vi "nanocal -- nuclear schottky fit V5.vi"() -> ()   [LabVIEW 2020] (continued)
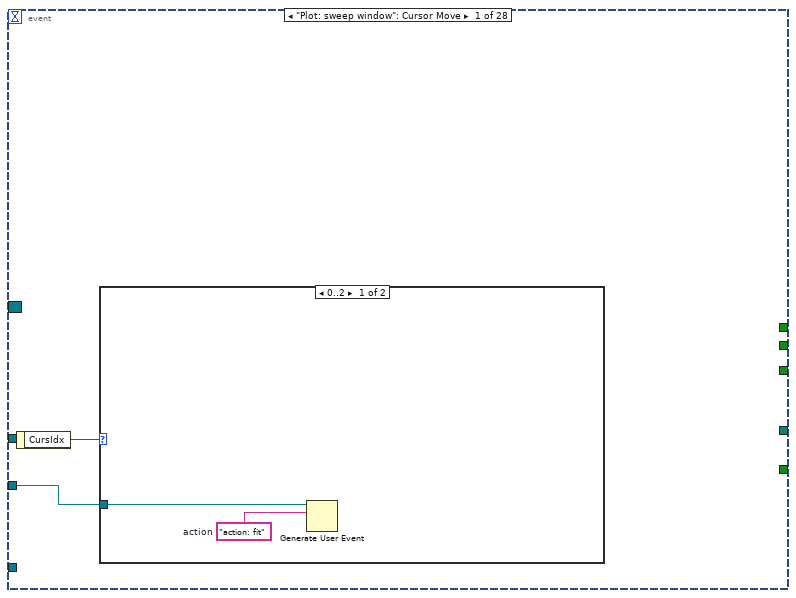
[diagram p2: hidden frame]
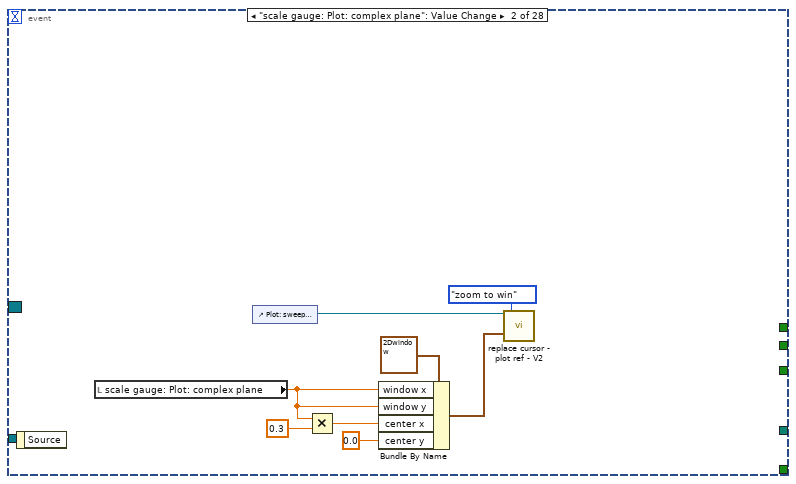
[diagram p4: hidden frame]
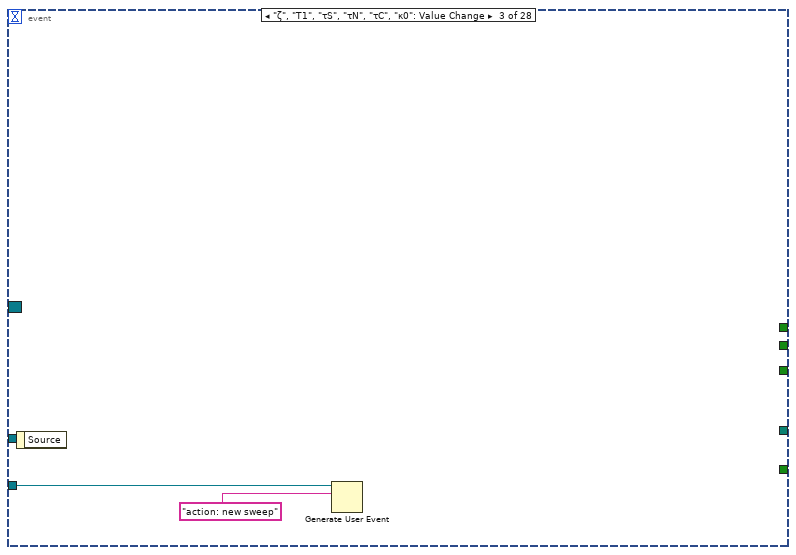
[diagram p5: hidden frame]
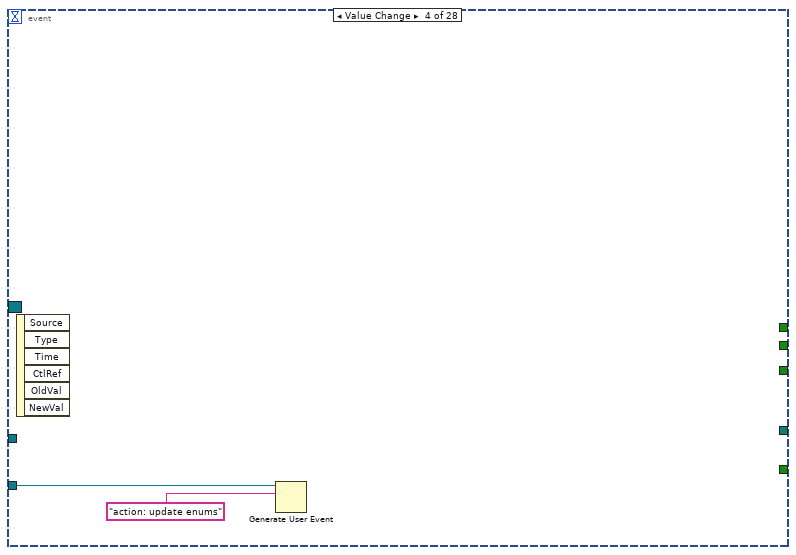
[diagram p6: hidden frame]
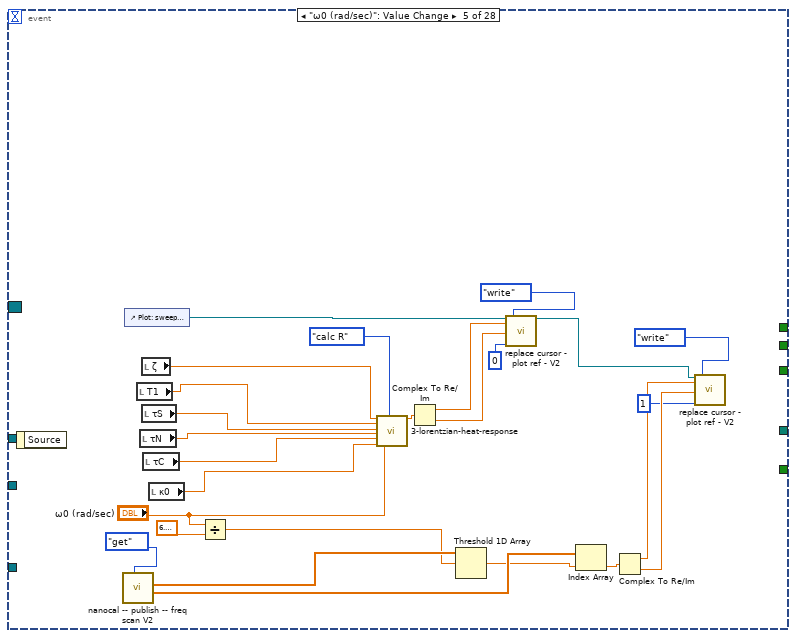
[diagram p7: hidden frame]
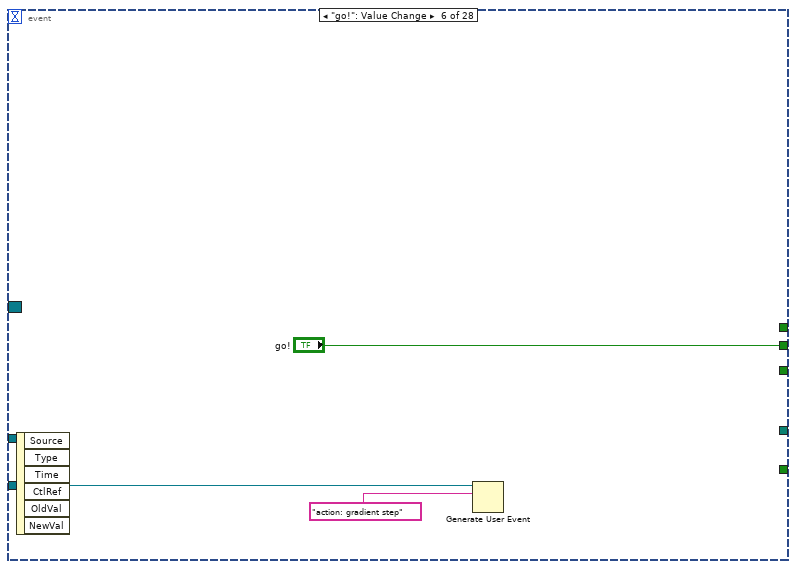
[diagram p8: hidden frame]
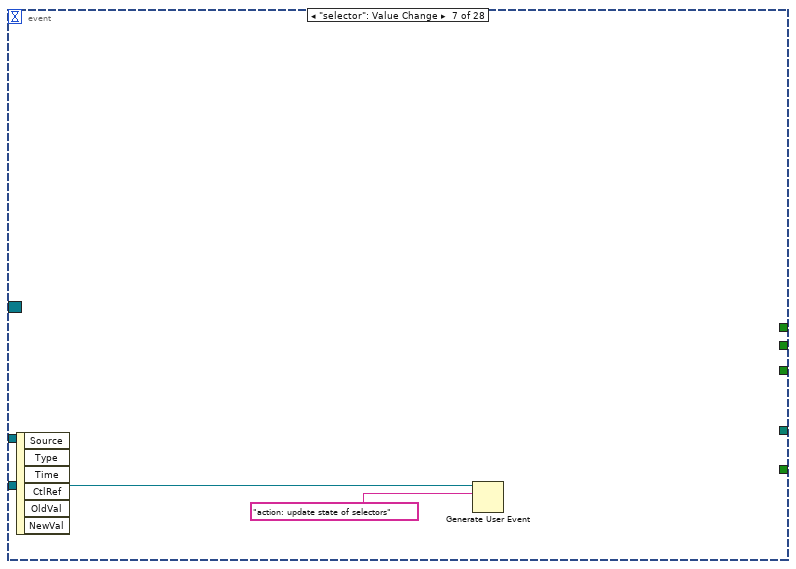
[diagram p9: hidden frame]
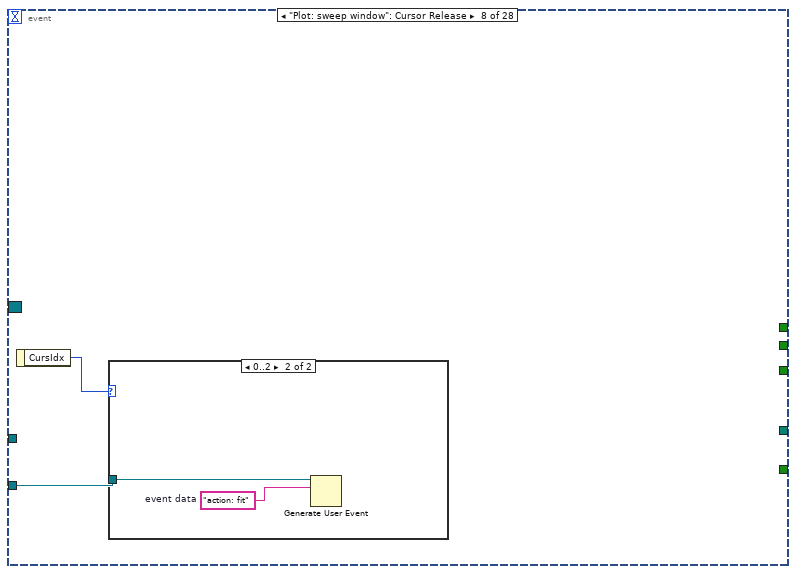
[diagram p10: hidden frame]
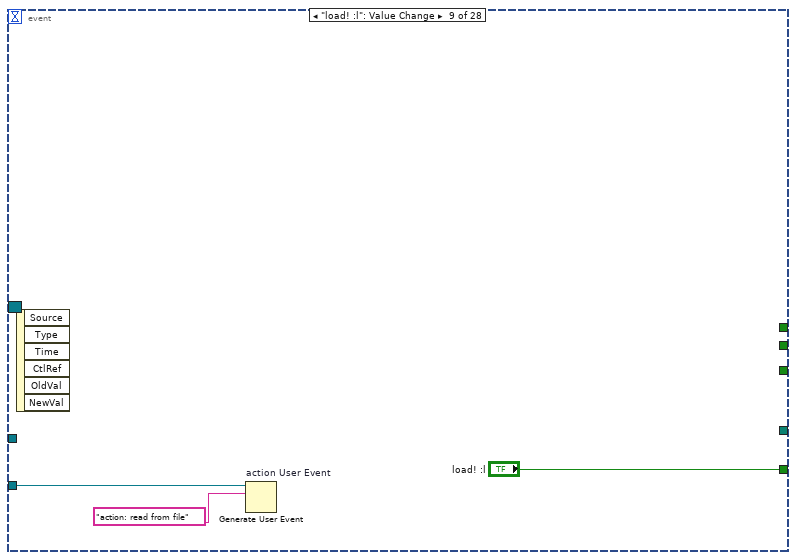
[diagram p12: hidden frame]
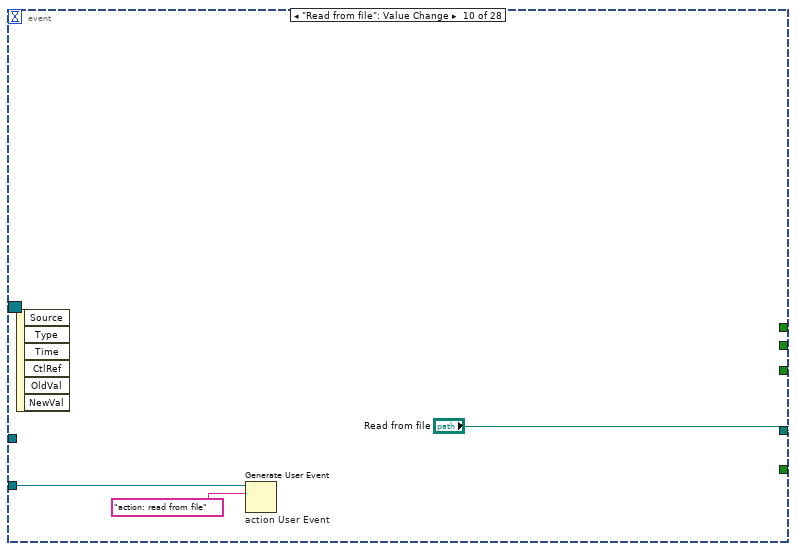
[diagram p13: hidden frame]
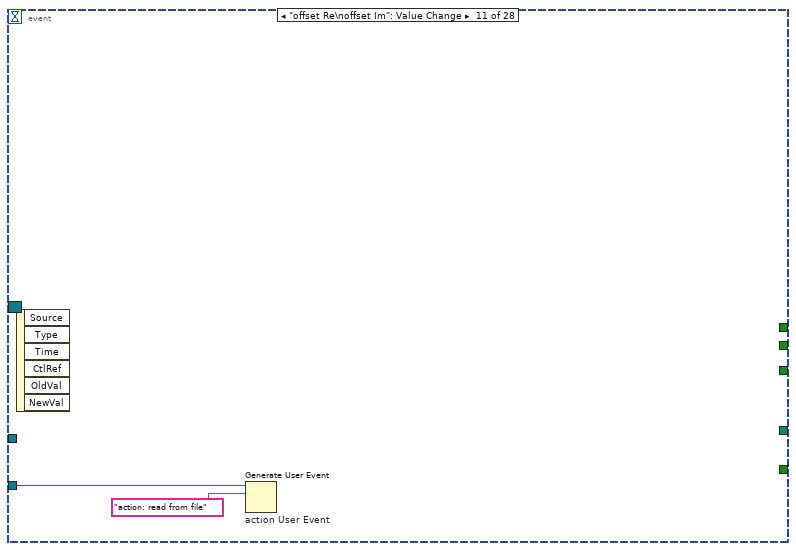
[diagram p14: hidden frame]
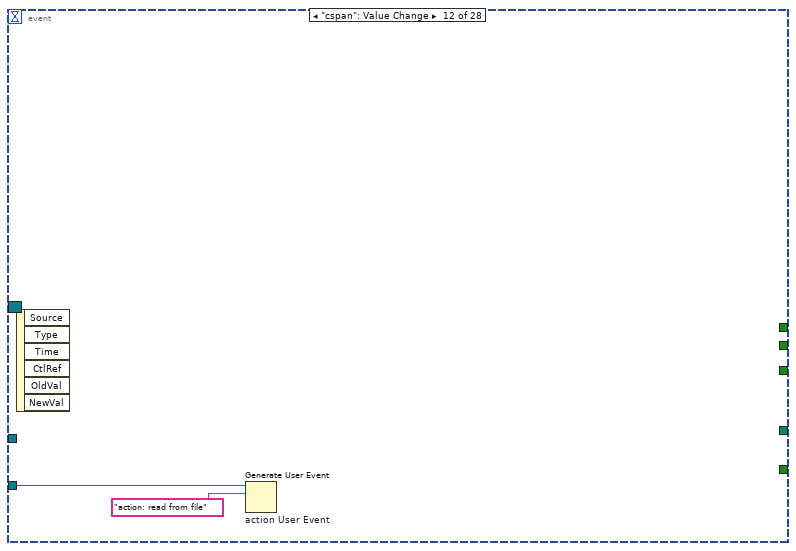
[diagram p15: hidden frame]
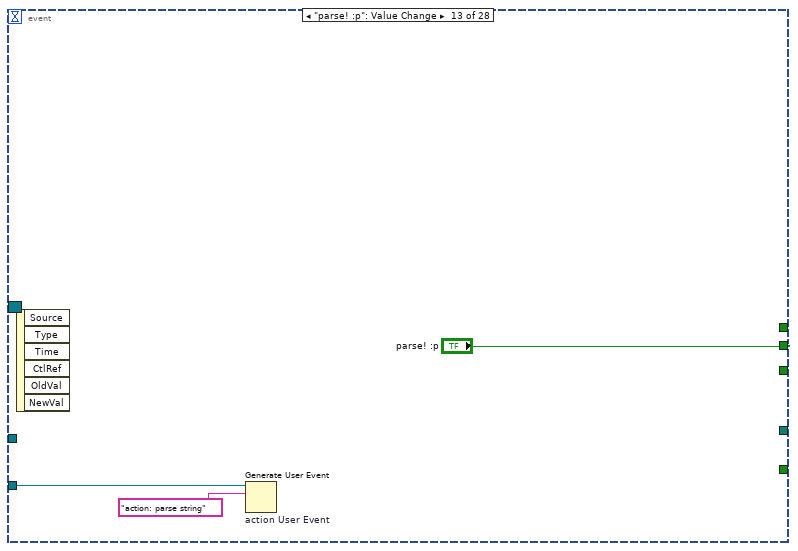
[diagram p16: hidden frame]
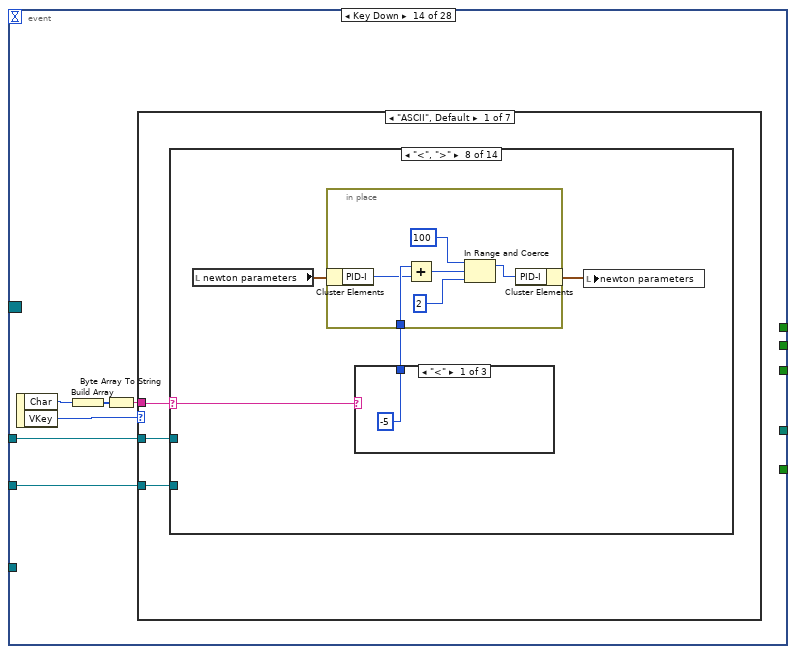
[diagram p17: hidden frame]
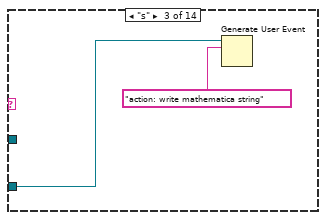
[diagram p20: hidden frame]
              frame "Up", Default {
              }
              frame "Down" {
              }
              frame "Left" {
              }
              frame "Right" {
              }
            }
            n720 = call "replace cursor - plot ref - V2.vi"("Plot ref in"=w1412, "cursor action"=w1414) -> ()  [unwired: 14 in, 4 out]
          }
        }
      }
      event "Plot:  colors": Cursor Move {
        n721 = event-data() -> ("CursIdx"=w1422:i32)  [unwired: 1 in]
        n722 = local read "τS"() -> (w1439:dbl)
        n723 = local read "τN"() -> (w1440:dbl)
        n724 = local read "τC"() -> (w1441:dbl)
        n725 = local read "T1"() -> (w1438:dbl)
        n726 = local read "κ0"() -> (w1442:dbl)
        n727 = local read "ζ"() -> (w1437:dbl)
        n728 = call "replace cursor - plot ref - V2.vi"("Plot ref in"=w1443, "cursor index"=w1422, "cursor action"=cursor_action."read") -> ("read Y"=w1421:dbl)  [unwired: 13 in, 3 out]
        n729 = Build Array(w1437, w1438, w1439, w1440, w1441, w1442) -> (w1424:dbl[])
        n730 = Replace Array Subset(array=w1424, new element=w1421, index=w1422) -> (w1423:dbl[])
        n731 = Index Array(array=w1423, index #1=0 ("index"), index #2=1 ("index"), index #3=2 ("index"), index #4=3 ("index"), index #5=4 ("index"), index #6=5 ("index")) -> (element #1=w1430:dbl, element #2=w1429:dbl, element #3=w1428:dbl, element #4=w1427:dbl, element #5=w1426:dbl, element #6=w1425:dbl)
        n732 = Generate User Event(user event=w1420, event data cluster="action: replot circles" ("event data")) -> ()  [unwired: 2 in, 2 out]
        n733 = local write "τN"(w1427) -> ()
        n734 = local write "τC"(w1426) -> ()
        n735 = local write "τS"(w1428) -> ()
        n736 = local write "κ0"(w1425) -> ()
        n737 = local write "T1"(w1429) -> ()
        n738 = local write "ζ"(w1430) -> ()
      }
      event "pause!": Value Change {
        n739 = event-data() -> ()  [unwired: 1 in, 6 out]
        n740 = local write "newton pause"(TRUE ("newton pause")) -> ()
      }
      event "uco! :u": Value Change {
        n741 = event-data() -> ()  [unwired: 1 in, 1 out]
        n742 = Generate User Event(user event=w1448, event data cluster="ignoreaction: uco" ("event data")) -> ()  [unwired: 2 in, 2 out]
      }
      event "Math→τ! :q": Value Change {
        n743 = event-data() -> ()  [unwired: 1 in, 1 out]
        n744 = Generate User Event(user event=w1451, event data cluster="action: copy from math" ("event data")) -> ()  [unwired: 2 in, 2 out]
      }
      event "load default values": Value Change {
        n745 = event-data() -> ()  [unwired: 1 in, 1 out]
        n746 = Generate User Event(user event=w1453, event data cluster="action: update default values" ("event data")) -> ()  [unwired: 2 in, 2 out]
      }
      event "τ→Math! :p": Value Change {
        n747 = event-data() -> ()  [unwired: 1 in, 1 out]
        n748 = Generate User Event(user event=w1457, event data cluster="action: copy to math" ("event data")) -> ()  [unwired: 2 in, 2 out]
      }
      event "Math→ string OUT! :s": Value Change {
        n749 = event-data() -> ()  [unwired: 1 in, 1 out]
        n750 = Generate User Event(user event=w1460, event data cluster="action: write mathematica string" ("event data")) -> ()  [unwired: 2 in, 2 out]
      }
      event "generate empty string from filelist !": Value Change {
        n751 = event-data() -> ()  [unwired: 1 in, 1 out]
        n752 = Generate User Event(user event=w1463, event data cluster="action: empty string from filelist" ("event data")) -> ()  [unwired: 2 in, 2 out]
      }
      event "string IN → Math!": Value Change {
        n753 = event-data() -> ()  [unwired: 1 in, 1 out]
        n754 = Generate User Event(user event=w1466, event data cluster="action: read mathematica string" ("event data")) -> ()  [unwired: 2 in, 2 out]
      }
      event "filenames": Value Change {
        n755 = event-data() -> ()  [unwired: 1 in, 6 out]
        n756 = local read "filesnames lookup"() -> (w1473:map{i32, string})
        n757 = local read "all full filenames"() -> (w1471:map{string, path})
        n758 = local read "filenames"() -> (w1472:u16)
        n759 = Look In Map(map=w1473, key=w1472) -> (value=w1470:string)  [unwired: 1 in, 1 out]
        n760 = Look In Map(map=w1471, key=w1470) -> (value=w1468:path)  [unwired: 1 in, 1 out]
        n761 = for {
          N: 1 -> [_]
          tunnel: w1474 -> [w1476]
          tunnel: w1468 -> [w1475]
          n762 = local write "Read from file"(w1475) -> ()
          n763 = Generate User Event(user event=w1476, event data cluster="action: read from file" ("event data")) -> ()  [unwired: 2 in, 2 out]
        }
      }
      event "selection :|\\": Value Change {
        n764 = event-data() -> ()  [unwired: 1 in, 6 out]
        n765 = Generate User Event(user event=w1478, event data cluster="action: constrained filenames select" ("event data")) -> ()  [unwired: 2 in, 2 out]
      }
      event User Event {
        n766 = event-data() -> ("interface"=w1481:string)  [unwired: 1 in, 4 out]
        n767 = case shown="\"interface: update color cursors\"" w1481 {
          tunnel: [_ _ TRUE] -> w1480
          frame "void", Default {
          }
          frame "interface: update color cursors" {
            w1485 = T1[] [enum."T (K)", enum."B (T)", enum."θ (deg)"] items=["ζ", "τ1", "τS", "τN", "τC", "κ0", "m1", "m2", "m3", "T (K)", "B (T)", "θ (deg)", "side (S|R)", "set of (B|T)", "Re(offset)", "Im(offset)"]
            w1482 = T1[] [enum."ζ", enum."τ1", enum."τS", enum."τN", enum."τC", enum."κ0", enum."m1", enum."m2", enum."m3"] items=["ζ", "τ1", "τS", "τN", "τC", "κ0", "m1", "m2", "m3", "T (K)", "B (T)", "θ (deg)", "side (S|R)", "set of (B|T)", "Re(offset)", "Im(offset)"]
            n768 = local read "τN"() -> (w1495:dbl)
            n769 = local read "τC"() -> (w1496:dbl)
            n770 = local read "T1"() -> (w1493:dbl)
            n771 = local read "κ0"() -> (w1497:dbl)
            n772 = local read "τS"() -> (w1494:dbl)
            n773 = local read "cursor x selector"() -> (w1488:map{T1, dbl})
            n774 = local read "ζ"() -> (w1492:dbl)
            n775 = local read "X selector"() -> (w1489:T1)
            n776 = local read "T (K)"() -> (w1490:dbl)
            n777 = Build Array(w1492, w1493, w1494, w1495, w1496, w1497) -> (w1499:dbl[])
            n778 = Look In Map(map=w1488, key=w1489, default value=w1490) -> (value=w1491:dbl)  [unwired: 1 out]
            n779 = for {
              shift-right: [w1515] -> w1500
              shift-left: map{T1, dbl} {} ("Map IN") -> [w1516]
              tunnel: w1482 -> [w1513] mode=indexing
              tunnel: w1499 -> [w1514] mode=indexing
              tunnel: [w1513] -> w1508 mode=indexing
              n780 = Insert Into Map(map in=w1516, key=w1513, value=w1514) -> (map out=w1515:map{T1, dbl})  [unwired: 2 out]
            }
            n781 = local read "cursor index map"() -> (w1498:map{T1, i32})
            n782 = local read "θ (deg)"() -> (w1503:dbl)
            n783 = local read "B (T)"() -> (w1502:dbl)
            n784 = local read "T (K)"() -> (w1501:dbl)
            n785 = Build Array(w1501, w1502, w1503) -> (w1505:dbl[])
            n786 = control-ref of="Plot:  colors"() -> (w1487:refnum<vi>)
            n787 = call "3-lorentzian-heat-response -- V4.vi"("action"=3-lorentzian-heat-response_action."calc m1m2m3", "Map IN"=w1500) -> ("Map OUT"=w1504:map{T1, dbl})  [unwired: 7 in, 2 out]
            n788 = for {
              shift-right: [w1511] -> w1506
              shift-left: w1504 -> [w1512]
              tunnel: w1485 -> [w1510] mode=indexing
              tunnel: w1505 -> [w1509] mode=indexing
              n789 = Insert Into Map(map in=w1512, key=w1510, value=w1509) -> (map out=w1511:map{T1, dbl})  [unwired: 2 out]
            }
            n790 = for {
              tunnel: w1491 -> [w1524]
              tunnel: w1487 -> [w1523]
              tunnel: w1508 -> [w1519] mode=indexing
              tunnel: w1498 -> [w1521]
              shift-right: [w1518] -> _
              shift-left: w1504 -> [w1518]
              n791 = Look In Map(map=w1518, key=w1519) -> (value=w1517:dbl)  [unwired: 1 in, 1 out]
              n792 = Look In Map(map=w1521, key=w1519) -> (value=w1520:i32)  [unwired: 1 in, 1 out]
              n793 = call "replace cursor - plot ref - V2.vi"("Plot ref in"=w1523, "new X"=w1524, "new  Y"=w1517, "cursor index"=w1520, "cursor action"=cursor_action."write") -> ()  [unwired: 11 in, 4 out]
            }
            n794 = call "string parse mathematica assosiated array.vi"("action"=mathematica_string_map_action."create string" ("derivative"), "map IN"=w1506) -> ("String OUT"=w1507:string)  [unwired: 8 in, 1 out]
            n795 = local write "String"(w1507) -> ()
          }
          frame "interface: exit" {
          }
        }
      }
      event "plot landscape!", "range one", "range two": Value Change {
        n796 = event-data() -> ()  [unwired: 1 in, 6 out]
        n797 = Generate User Event(user event=w1526, event data cluster="action: plot landscape" ("event data")) -> ()  [unwired: 2 in, 2 out]
      }
      event "colors": Value Change {
        n798 = event-data() -> ()  [unwired: 1 in, 6 out]
        n799 = Generate User Event(user event=w1529, event data cluster="action: reset colors" ("event data")) -> ()  [unwired: 2 in, 2 out]
      }
    }
  }
  "cursor x selector" <- w18
